vi "RIOGlobal.vi"() -> ()   [LabVIEW 2015]
panel:
  out "T PWM rev":dbl=68.375
  out "VS_TCU +-":dbl
  out "Current RMS":dbl=25.0 format="%0.2f"
  out "sol_temp":bool=TRUE
  out "VS_saved":dbl
  out "Encoder percent":dbl=84.3595
  in  "Current lmt":dbl=25.0 format="%0.2f"
  out "amp_ini":dbl=2.501611328125 format="%.13g"
  out "B ts":u32=5
  in  "Encoder 100":dbl=150.793
  in  "Encoder 0":dbl=236.559
  out "T PWM Ini":dbl=6223.0
  out "T PWM":dbl=68.375
  out "Throttle_Enable":bool=TRUE
  out "B Push percent":dbl
  out "Brake_Act":bool
  in  "B PWM Min":dbl=-80.0
  in  "B PWM Max":dbl=80.0
  out "B PWM":dbl=-100.0
  out "T Lim":bool=TRUE
  out "Encoder":dbl=84.3595
  out "Auto":bool
  out "Run":bool
  out "SAS_angle_MDPS":dbl=-1.03271484375
  out "Can_ini":bool
  out "rpm":dbl=655.5
  out "G_sel_disp":u8
  out "MDPS_Control":dbl=-0.0
  out "VS_Desire":dbl=1.0
  out "TPS":dbl
  out "VS_TCU":dbl
  out "throttle control input":dbl=18.374999999999996
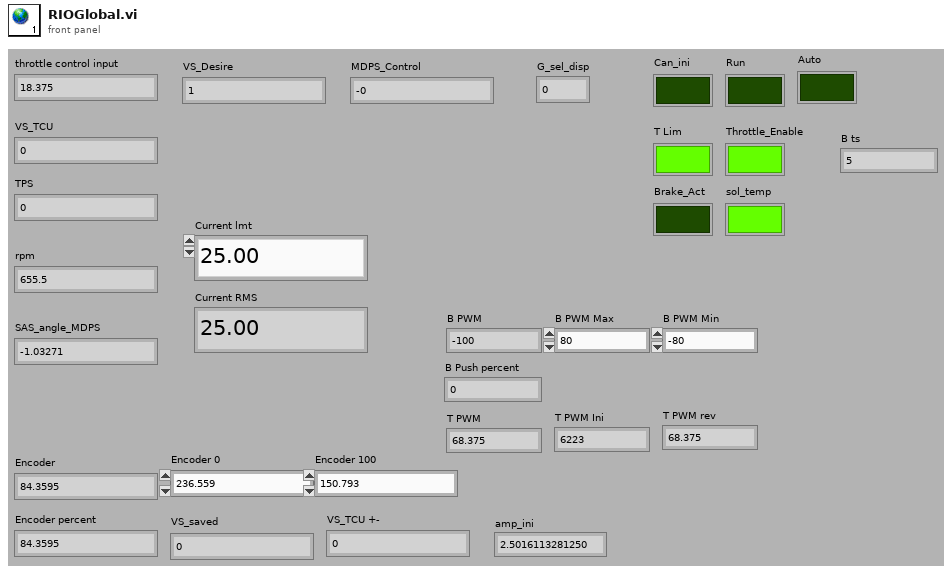
[diagram p1: front panel]
diagram:
